vi "3.2.vi"() -> ()   [LabVIEW 2020]
panel:
  in  "Numeric 2":dbl
  in  "Numeric":dbl
  out "XY Graph":cluster{dbl[], dbl[]}(graph)
  out "Phi":dbl[](array[numeric])
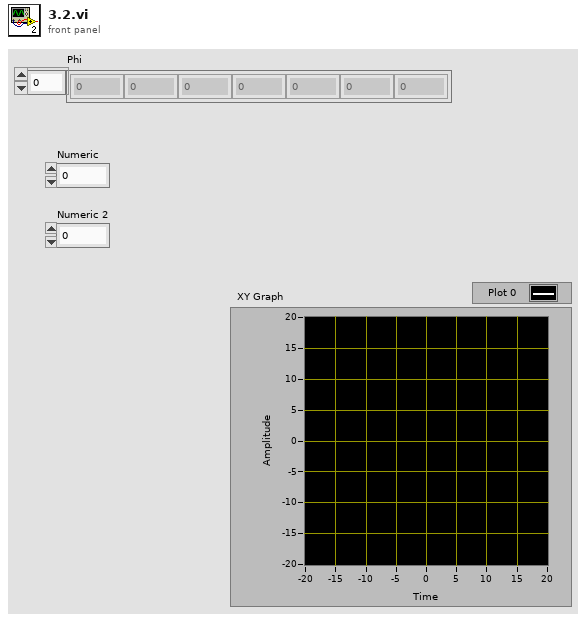
[diagram p1: front panel]
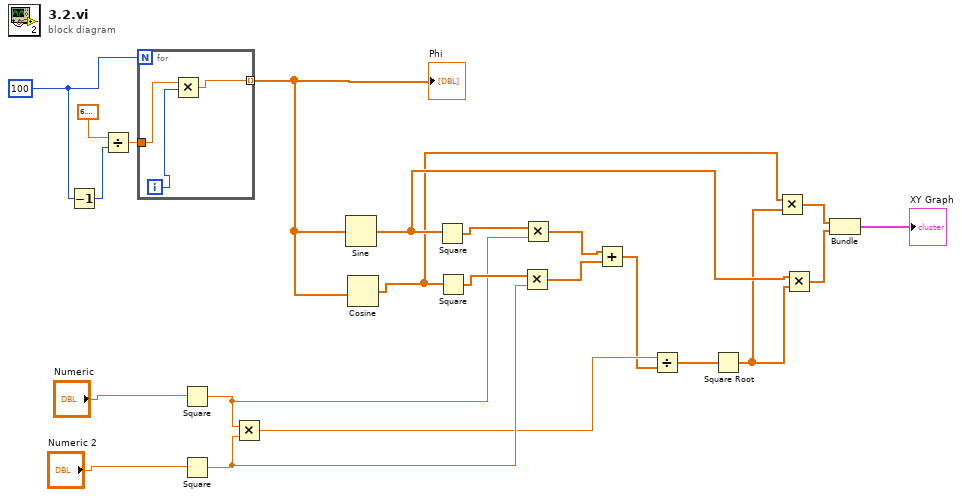
[diagram p0: block diagram]
diagram:
  w21 = 100
  n1 = Decrement(x=w21) -> (x-1=w20:i32)
  n2 = Divide(x=6.283185307179586, y=w20) -> (x/y=w19:dbl)
  n3 = for {
    N: w21 -> [_]
    tunnel: w19 -> [w25]
    tunnel: [w23] -> w17 mode=indexing
    i -> [w24]
    n4 = Multiply(x=w25, y=w24) -> (x*y=w23:dbl)
  }
  "Phi" <- w17
  n5 = Square(x="Numeric") -> (x^2=w14:dbl)
  n6 = Square(x="Numeric 2") -> (x^2=w13:dbl)
  n7 = Multiply(x=w14, y=w13) -> (x*y=w10:dbl)
  n8 = Sine(x=w17) -> (sin(x)=w7:dbl[])
  n9 = Cosine(x=w17) -> (cos(x)=w5:dbl[])
  n10 = Square(x=w7) -> (x^2=w16:dbl[])
  n11 = Square(x=w5) -> (x^2=w15:dbl[])
  n12 = Multiply(x=w15, y=w13) -> (x*y=w11:dbl[])
  n13 = Multiply(x=w16, y=w14) -> (x*y=w12:dbl[])
  n14 = Add(x=w12, y=w11) -> (x+y=w9:dbl[])
  n15 = Divide(x=w10, y=w9) -> (x/y=w8:dbl[])
  n16 = Square Root(x=w8) -> (sqrt(x)=w6:dbl[])
  n17 = Multiply(x=w5, y=w6) -> (x*y=w4:dbl[])
  n18 = Multiply(x=w7, y=w6) -> (x*y=w3:dbl[])
  n19 = Bundle "Bundle"(w4, w3) -> (→"XY Graph":cluster{dbl[], dbl[]})  [unwired: 1 in]
